vi "RSZVB Get Pulse Evaluation Section Stop.vi"(5 "Record Number (1)":i32=1, 6 "Generator/Port Number (1)":i32=1, 7 "Interface Type (0: Generator)":i32(ring) items=["Generator", "Analyzer Source"], 8 "error in (no error)":errorcluster {"code" format="%.0x"}, 9 "Receiver Type (0: A)":i32(ring) items=["A", "B"], 10 "Channel (1)":i32=1, 11 "VISA session":refnum<visa-resource-name>) -> (0 "error out":errorcluster {"code" format="%.0x"}, 1 "Evaluation Stop Time":dbl format="%^.3e", 3 "dup VISA session":refnum<visa-resource-name>)   [LabVIEW 2011]
doc: "This VI returns the stop time of the averaging section for the wave quantity.\n\nRemote-control command(s):\n[SENSe<Ch>:]PULSe:RECeiver:A<rec_no>:GENerator<gen_no>:EVALuation:STOP?\n[SENSe<Ch>:]PULSe:RECeiver:A<rec_no>:SRCPort<port_no>:EVALuation:STOP?\n[SENSe<Ch>:]PULSe:RECeiver:B<rec_no>:GENerator<gen_no>:EVALuation:STOP?\n[SENSe<Ch>:]PULSe:RECeiver:B<rec_no>:SRCPort<port_no>:EVALuation:STOP?"
uses:
  _utility/RSZVB Global Data.vi
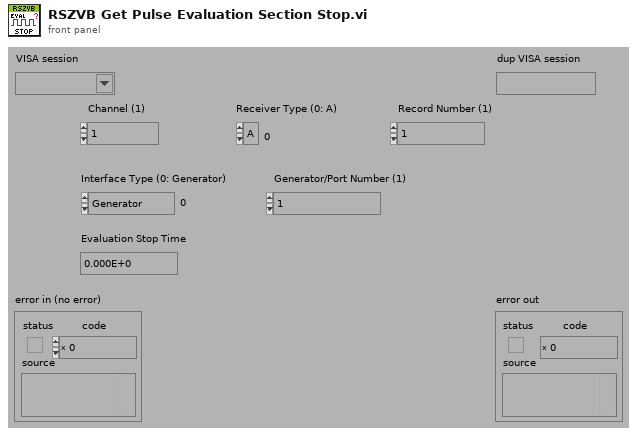
[diagram p1: front panel]
types:
  T1 = cluster{"Error Checking (T: On)":bool, "Installed Options":string[], "Data Valid?":bool, "Ports":i32, "Model":string[], "Option Checking (T: On)":bool}[]
  T2 = cluster{"Error Checking (T: On)":bool, "Installed Options":string[], "Data Valid?":bool, "Ports":i32, "Model":string[], "Option Checking (T: On)":bool}
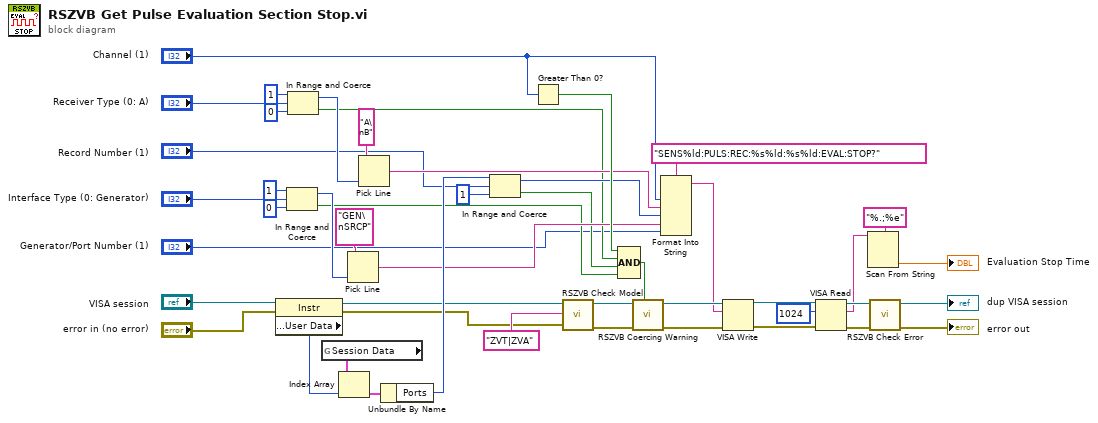
[diagram p0: block diagram]
diagram:
  n1 = property class="Instr"(reference="VISA session", error in="error in (no error)") -> (reference out=w26:refnum<visa-resource-name>, error out=w25:errorcluster, "General Settings:User Data"=w28:u32)
  n2 = In Range and Coerce(upper limit=1, x="Interface Type (0: Generator)", lower limit=0) -> (coerced(x)=w31:i32, In Range?=w18:bool)
  n3 = In Range and Coerce(upper limit=1, x="Receiver Type (0: A)", lower limit=0) -> (coerced(x)=w35:i32, In Range?=w20:bool)
  n4 = global read "RSZVB Global Data.vi" "Session Data"() -> (w29:T1)
  n5 = Index Array(array=w29, index=w28) -> (element=w30:T2)
  n6 = Pick Line(multi-line string="GEN\nSRCP", line index=w31) -> (output string=w21:string)  [unwired: 1 in]
  n7 = Pick Line(multi-line string="A\nB", line index=w35) -> (output string=w23:string)  [unwired: 1 in]
  n8 = Unbundle By Name(w30) -> ("Ports"=w27:i32)
  n9 = In Range and Coerce(upper limit=w27, x="Record Number (1)", lower limit=1) -> (coerced(x)=w22:i32, In Range?=w19:bool)
  n10 = Greater Than 0?(x="Channel (1)") -> (x > 0?=w42:bool)
  n11 = call "RSZVB Check Model.vi"("error in (no error)"=w25, "Model"="ZVT|ZVA" ("Options"), "VISA session"=w26) -> ("error out"=w40:errorcluster, "dup VISA session"=w39:refnum<visa-resource-name>)  [unwired: 7 in]
  n12 = Compound Arithmetic op=AND(w42, w20, w19, w18) -> (w44:bool)
  n13 = call "RSZVB Coercing Warning.vi"("In Range?"=w44, "error in (no error)"=w40, "VISA session"=w39) -> ("error out"=w45:errorcluster, "dup VISA session"=w46:refnum<visa-resource-name>)  [unwired: 7 in]
  n14 = Format Into String(format string="SENS%ld:PULS:REC:%s%ld:%s%ld:EVAL:STOP?", "Channel (1)", w23, w22, w21, "Generator/Port Number (1)") -> (resulting string=w43:string)  [unwired: 2 in, 1 out]
  n15 = VISA Write(VISA resource name=w46, write buffer=w43, error in (no error)=w45) -> (VISA resource name out=w11:refnum<visa-resource-name>, error out=w12:errorcluster)  [unwired: 1 out]
  n16 = VISA Read(VISA resource name=w11, byte count=u32 1024 ("byte count (0)"), error in (no error)=w12) -> (VISA resource name out=w16:refnum<visa-resource-name>, read buffer=w13:string, error out=w15:errorcluster)  [unwired: 1 out]
  n17 = Scan From String(format string="%.;%e", input string=w13) -> (output 1=→"Evaluation Stop Time":dbl)  [unwired: 3 in, 3 out]
  n18 = call "RSZVB Check Error.vi"("error in (no error)"=w15, "VISA session"=w16) -> ("error out"=→"error out":errorcluster, "dup VISA session"=→"dup VISA session":refnum<visa-resource-name>)  [unwired: 8 in]
